vi "Actor Core.vi"(8 "error in":errorcluster, 11 "Message Logger in":refnum<class "Classic Logger.lvclass">) -> (0 "error out":errorcluster, 3 "Actor out":refnum<class "Actor.lvclass">)   [LabVIEW 2023, in "Monitored Actor.lvlib" / "Classic Logger.lvclass"]
doc: "(<B>Filename</B>: Actor Framework.lvlib:Actor.lvclass:Actor Core.vi)\n\nReceives messages to the actor, reacts to them, and initiates any error handling that may shut the actor down.\n\nDescendant classes may override this VI to append parallel tasks for the actor to complete while it handles messages. Overrides use the Call Parent Method node."
uses:
  Classic Logger.lvclass
  C:/Users/Public/Documents/Development/builds/Engine/Actor Framework.lvlibp/1abvi3w/vi.lib/ActorFramework/Actor/Actor.lvclass
  builds/Engine/Actor Framework.lvlibp/1abvi3w/vi.lib/ActorFramework/Actor/Actor.lvclass
  UI Data.ctl
  builds/Engine/Actor Framework.lvlibp/1abvi3w/vi.lib/ActorFramework/Message Enqueuer/Message Enqueuer.lvclass
  <vilib>/Utility/miscctls.llb/LVRowAndColumnTypeDef.ctl
  Classic Logger.lvclass/Classic Logger.ctl
  Monitor Data.ctl
  <vilib>/Utility/miscctls.llb/LVRowAndColumnUnsignedTypeDef.ctl
  Classic Logger Messages/Clear Log Msg/Clear Log Msg.lvclass
  Classic Logger Messages/Stop Logging Msg/Stop Logging Msg.lvclass
  builds/Engine/Actor Framework.lvlibp/1abvi3w/vi.lib/ActorFramework/Stop Msg/Stop Msg.lvclass
panel:
  in  "Actors":i32(listbox) caption="Actors Being Logged"
  in  "Stop Monitoring":bool
  in  "Log":i32(listbox)
  out "Filtered Msgs":i16
  in  "Clear Log":bool
  out "Message XML":string
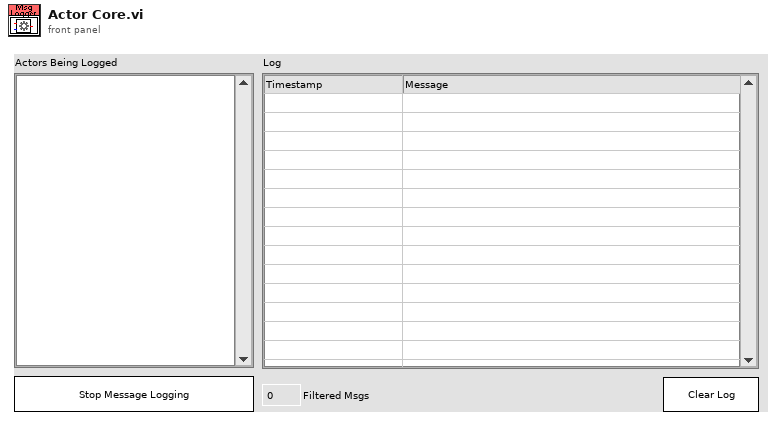
[diagram p1: front panel]
types:
  T1 = typedef "LVRowAndColumnTypeDef.ctl" = cluster{"Row":i32, "Column":i32}
  T2 = enum32{"Invalid", "Standard", "Closed", "Hidden", "Minimized", "Maximized"}
  T3 = typedef "Monitored Actor.lvlib/Classic Logger.lvclass/UI Data.ctl" = cluster{"Actors":cluster{"Q":refnum<class "Message Enqueuer.lvclass">, "Label":string}[], "Message Log":variant}
  T4 = typedef "LVRowAndColumnUnsignedTypeDef.ctl" = cluster{"Row":u32, "Column":u32}
  T5 = typedef "Monitored Actor.lvlib/Classic Logger.lvclass/Monitor Data.ctl" = cluster{"Time Stamp":timestamp, "class name":string, "Msg XML":string}
  T6 = cluster{"Q":refnum<class "Message Enqueuer.lvclass">, "Label":string}[]
  T7 = cluster{"Q":refnum<class "Message Enqueuer.lvclass">, "Label":string}
  T8 = cluster{"Actors":cluster{"Q":refnum<class "Message Enqueuer.lvclass">, "Label":string}[], "Message Log":variant}
  T9 = typedef "LVPoint32TypeDef.ctl" = cluster{"Horizontal":i32, "Vertical":i32}
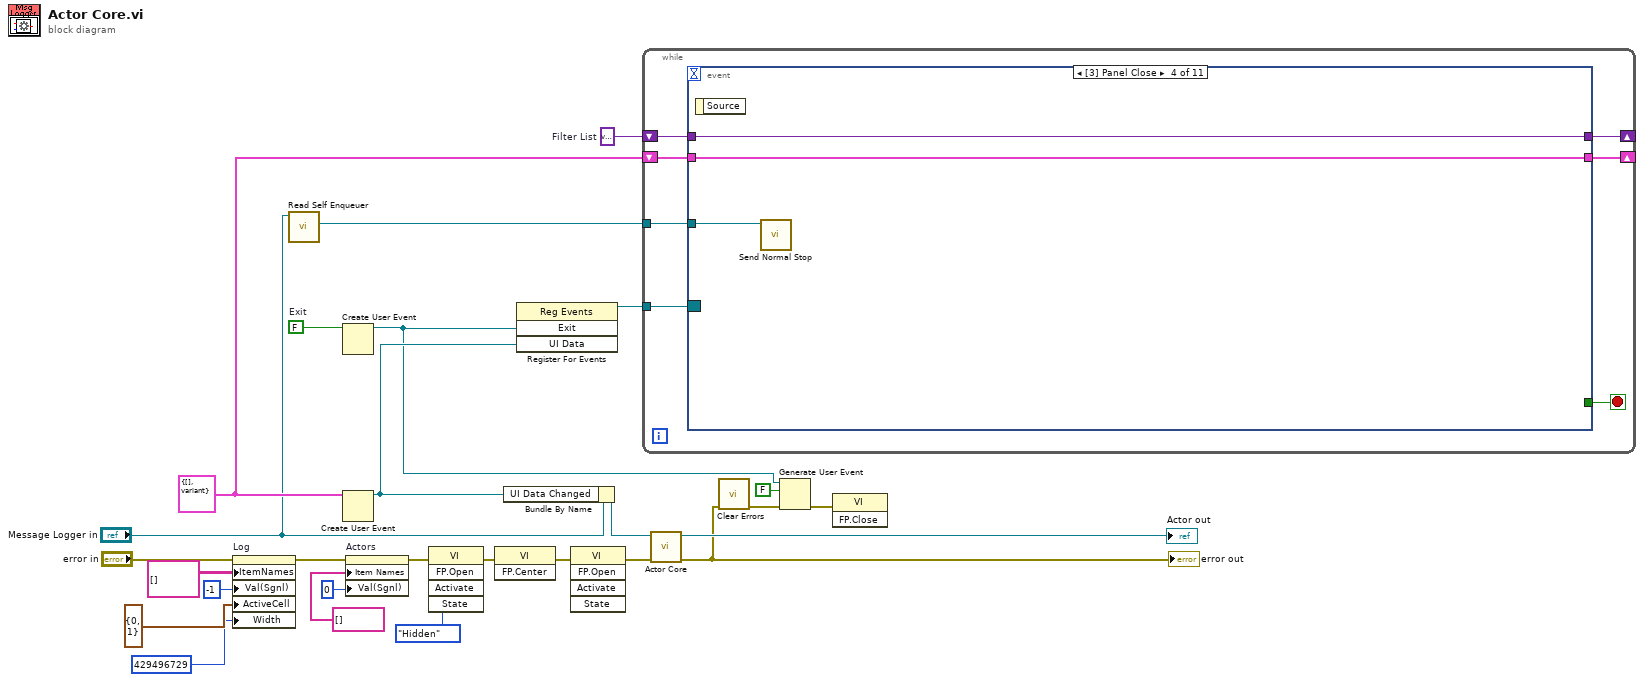
[diagram p0: block diagram]
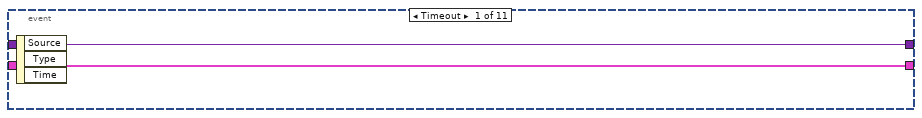
[diagram p2: hidden frame]
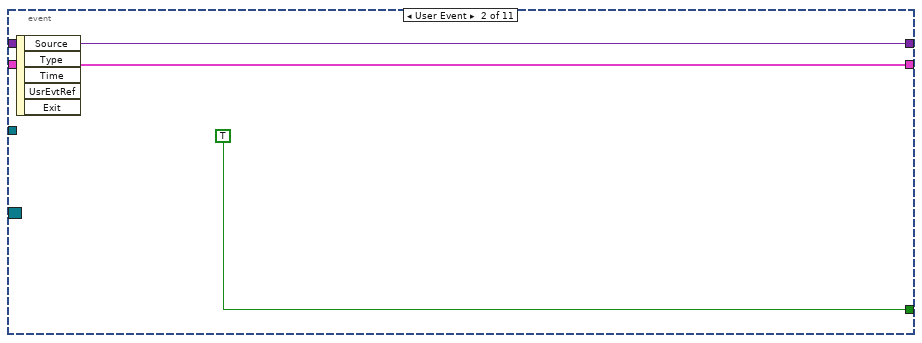
[diagram p3: hidden frame]
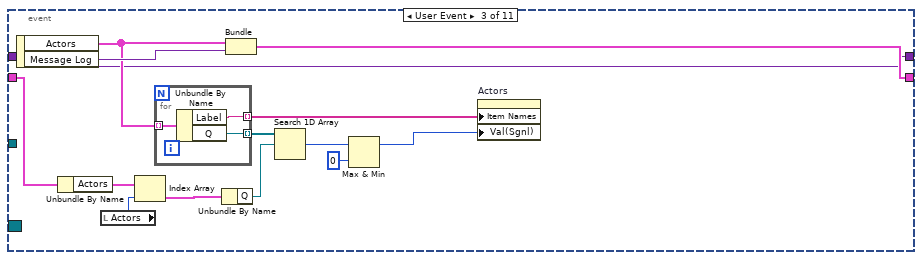
[diagram p4: hidden frame]
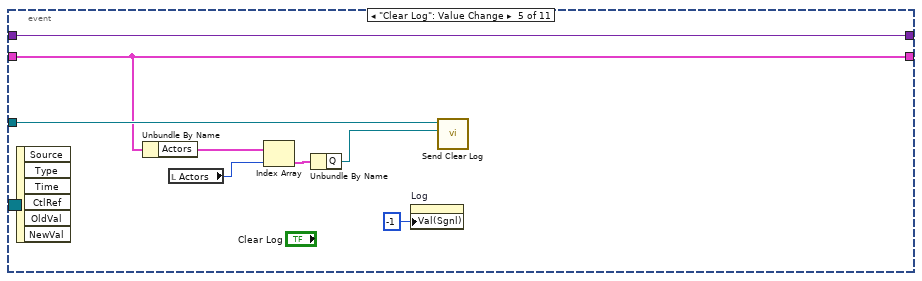
[diagram p5: hidden frame]
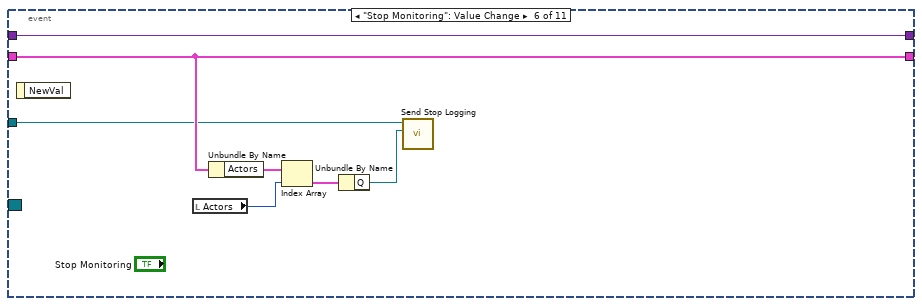
[diagram p6: hidden frame]
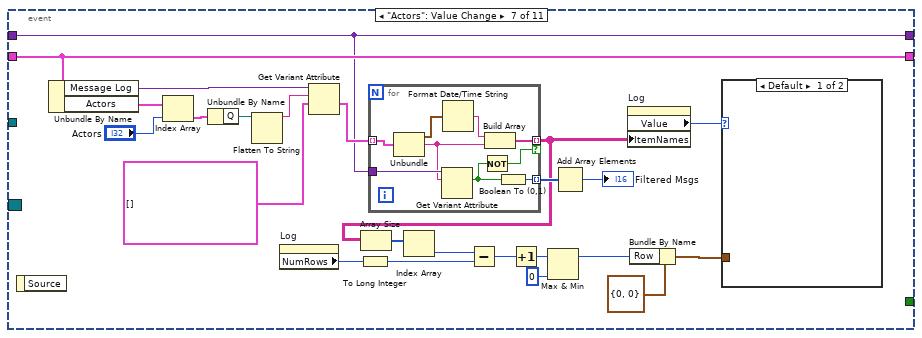
[diagram p7: hidden frame]
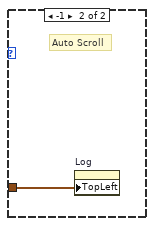
[diagram p8: hidden frame]
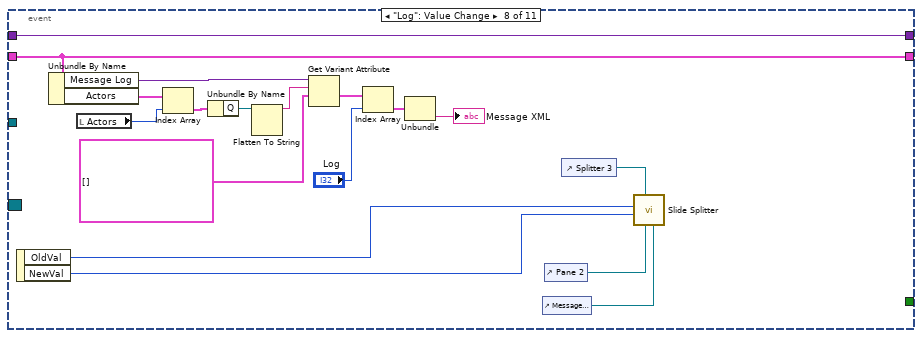
[diagram p9: hidden frame]
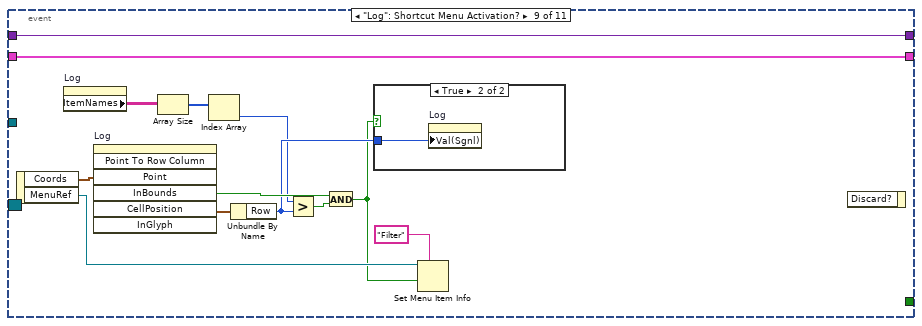
[diagram p10: hidden frame]
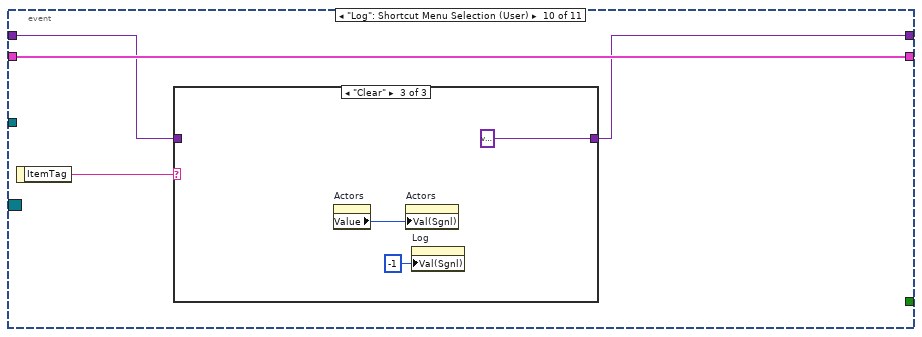
[diagram p12: hidden frame]
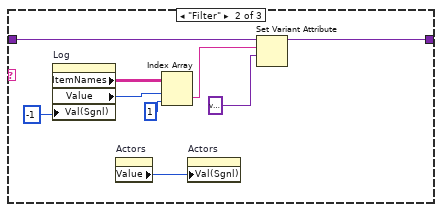
[diagram p14: hidden frame]
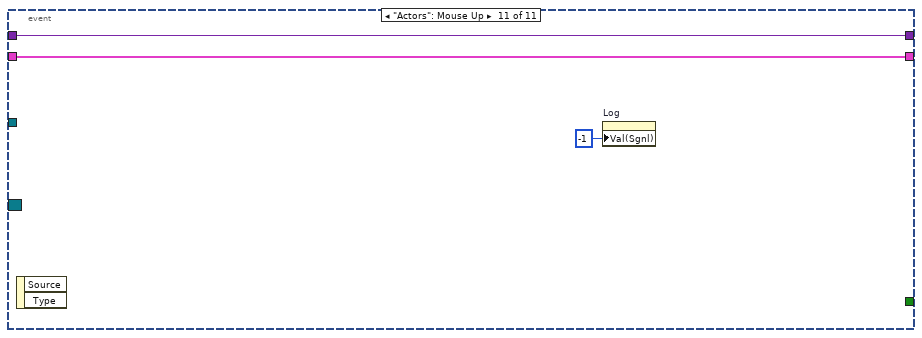
[diagram p15: hidden frame]
diagram:
  w5 = variant  # Filter List
  w21 = FALSE  # Exit
  w13 = T3 {"Actors"=[], "Message Log"=variant} ("UI Data")
  n1 = property on="Log" class="MCListbox (strict)"(error in="error in", "ItemNames"=string[][] [] ("Item Names"), "Val(Sgnl)"=-1 ("Log"), "ActiveCell"=T1 {"Row"=0, "Column"=1} ("Active Cell:Active Cell"), "Width"=u32 429496729 ("Active Cell:Cell Size:Width")) -> (error out=w15:errorcluster)  [unwired: 1 in, 1 out]
  n2 = call "Read Self Enqueuer.vi"("Actor"="Message Logger in") -> ("Self Enqueuer"=w11:refnum<class "Message Enqueuer.lvclass">)  [unwired: 10 in]
  n3 = Create User Event(user event datatype=w21) -> (user event=w18:refnum<user-event>)  [unwired: 1 in, 1 out]
  n4 = Create User Event(user event datatype=w13) -> (user event=w23:refnum<user-event>)  [unwired: 1 in, 1 out]
  n5 = property on="Actors" class="LstBox (strict)"(error in=w15, "Item Names"=string[] [], "Val(Sgnl)"=0 ("Log")) -> (error out=w9:errorcluster)  [unwired: 1 in, 1 out]
  n6 = invoke class="VI" method="FP.Open"(error in=w9, "State"=T2."Hidden") -> (error out=w8:errorcluster)  [unwired: 3 in, 4 out]
  n7 = invoke class="VI" method="FP.Center"(error in=w8) -> (error out=w7:errorcluster)  [unwired: 2 in, 2 out]
  n8 = Bundle By Name(cluster="Message Logger in", "UI Data Changed"=w23) -> (w24:refnum<class "Classic Logger.lvclass">)
  n9 = register-events(w18, w23) -> (reference out=w22:refnum<event-registration>)  [unwired: 2 in, 1 out]
  n10 = invoke class="VI" method="FP.Open"(error in=w7) -> (error out=w17:errorcluster)  [unwired: 4 in, 4 out]
  n11 = while {
    tunnel: w22 -> [w34]
    shift-right: [w31] -> _
    shift-left: w13 -> [w32]
    tunnel: w11 -> [w30]
    shift-right: [w28] -> _
    shift-left: w5 -> [w29]
    stop <- w33 stop-if-true
    n12 = event shown="[3] Panel Close" {
      selector: w34 -> [_ _ _ _ _ _ _ _ _ _ _]
      dyn-events: _ -> [_ _ _ _ _ _ _ _ _ _ _]
      timeout: _ -> [_ _ _ _ _ _ _ _ _ _ _]
      tunnel: [_ TRUE _ _ _ _ _ _ _ _ _] -> w33
      tunnel: w32 -> [w36 w38 w47 w59 w66 w74 w98 w126 w137 w144 w160]
      tunnel: [w36 w38 w53 w59 w66 w74 w98 w126 w137 w144 w160] -> w31
      tunnel: w30 -> [_ _ _ w58 w67 w69 _ _ _ _ _]
      tunnel: w29 -> [w35 w37 w40 w57 w60 w70 w80 w114 w139 w142 w159]
      tunnel: [w35 w37 w40 w57 w60 w70 w80 w114 w139 w141 w159] -> w28
      event Timeout {
        n13 = event-data() -> ()  [unwired: 1 in, 3 out]
      }
      event User Event {
        n14 = event-data() -> ()  [unwired: 1 in, 5 out]
      }
      event User Event {
        n15 = event-data() -> ("Actors"=w51:T6, "Message Log"=w52:variant)  [unwired: 1 in]
        n16 = Unbundle By Name(w47) -> ("Actors"=w46:T6)
        n17 = local read "Actors"() -> (w45:i32)
        n18 = Index Array(array=w46, index=w45) -> (element=w44:T7)
        n19 = for {
          tunnel: w51 -> [w56] mode=indexing
          tunnel: [w55] -> w50 mode=indexing
          tunnel: [w54] -> w49 mode=indexing
          n20 = Unbundle By Name(w56) -> ("Label"=w55:string, "Q"=w54:refnum<class "Message Enqueuer.lvclass">)
        }
        n21 = Unbundle By Name(w44) -> ("Q"=w43:refnum<class "Message Enqueuer.lvclass">)
        n22 = Bundle("Actors"=w51, "Message Log"=w52) -> (w53:T8)  [unwired: 1 in]
        n23 = Search 1D Array(1D array=w49, element=w43) -> (index of element=w48:i32)  [unwired: 1 in]
        n24 = Max & Min(x=w48, y=0) -> (max(x,y)=w42:i32)  [unwired: 1 out]
        n25 = property on="Actors" class="LstBox (strict)"("Item Names"=w50, "Val(Sgnl)"=w42) -> ()  [unwired: 2 in, 2 out]
      }
      event Panel Close {
        n26 = event-data() -> ()  [unwired: 1 in, 1 out]
        n27 = call "Send Normal Stop.vi"("Message Enqueuer"=w58) -> ()  [unwired: 10 in, 1 out]
      }
      event "Clear Log": Value Change {
        n28 = event-data() -> ()  [unwired: 1 in, 6 out]
        n29 = Unbundle By Name(w66) -> ("Actors"=w65:T6)
        n30 = local read "Actors"() -> (w62:i32)
        n31 = Index Array(array=w65, index=w62) -> (element=w64:T7)
        n32 = Unbundle By Name(w64) -> ("Q"=w63:refnum<class "Message Enqueuer.lvclass">)
        n33 = property on="Log" class="MCListbox (strict)"("Val(Sgnl)"=-1 ("Value (Signaling)")) -> ()  [unwired: 2 in, 2 out]
        n34 = call "Send Clear Log.vi"("Actor Q"=w63, "Message Enqueuer in"=w67) -> ()  [unwired: 8 in, 2 out]
      }
      event "Stop Monitoring": Value Change {
        n35 = event-data() -> ()  [unwired: 1 in, 1 out]
        n36 = local read "Actors"() -> (w72:i32)
        n37 = Unbundle By Name(w74) -> ("Actors"=w73:T6)
        n38 = Index Array(array=w73, index=w72) -> (element=w71:T7)
        n39 = Unbundle By Name(w71) -> ("Q"=w68:refnum<class "Message Enqueuer.lvclass">)
        n40 = call "Send Stop Logging.vi"("Q"=w68, "Message Enqueuer in"=w69) -> ()  [unwired: 8 in, 2 out]
      }
      event "Actors": Value Change {
        n41 = event-data() -> ()  [unwired: 1 in, 1 out]
        n42 = Unbundle By Name(w98) -> ("Message Log"=w95:variant, "Actors"=w97:T6)
        n43 = Index Array(array=w97, index="Actors") -> (element=w94:T7)
        n44 = Unbundle By Name(w94) -> ("Q"=w91:refnum<class "Message Enqueuer.lvclass">)
        n45 = Flatten To String(anything=w91) -> (data string=w93:string)  [unwired: 3 in, 2 out]
        n46 = property on="Log" class="MCListbox (strict)"() -> ("NumRows"=w88:u32)  [unwired: 2 in, 2 out]
        n47 = Get Variant Attribute(Variant=w95, name=w93, default value (empty Variant)=T5[] []) -> (value=w90:T5[])  [unwired: 1 in, 3 out]
        n48 = To Long Integer(number=w88) -> (32bit integer=w81:i32)
        n49 = for {
          tunnel: w90 -> [w108] mode=indexing
          tunnel: [w105] -> w77 mode=indexing if=w102
          tunnel: w80 -> [w104]
          tunnel: [w100] -> w78 mode=indexing
          n50 = Unbundle(w108) -> ("Time Stamp"=w107:timestamp, "class name"=w103:string)  [unwired: 1 out]
          n51 = Get Variant Attribute(Variant=w104, name=w103) -> (found=w101:bool)  [unwired: 2 in, 3 out]
          n52 = Format Date/Time String(seconds (now)=w107) -> (date/time string=w106:string)  [unwired: 2 in]
          n53 = Not(x=w101) -> (.not. x?=w102:bool)
          n54 = Build Array(w106, w103) -> (w105:string[])
          n55 = Boolean To (0,1)(Boolean=w101) -> (0, 1=w100:i16)
        }
        n56 = Array Size(array=w77) -> (size(s)=w89:i32[])
        n57 = Index Array(array=w89) -> (element=w76:i32)  [unwired: 1 in]
        n58 = Subtract(x=w76, y=w81) -> (x-y=w86:i32)
        n59 = Increment(x=w86) -> (x+1=w85:i32)
        n60 = Max & Min(x=w85, y=0) -> (max(x,y)=w83:i32)  [unwired: 1 out]
        n61 = Add Array Elements(numeric array=w78) -> (sum=→"Filtered Msgs":i16)
        n62 = property on="Log" class="MCListbox (strict)"("ItemNames"=w77) -> ("Value"=w75:i32)  [unwired: 2 in, 2 out]
        n63 = Bundle By Name(cluster=T4 {"Row"=0, "Column"=0} ("Top Left Visible Cell"), "Row"=w83) -> (w84:T4)
        n64 = case shown="Default" w75 {
          tunnel: w84 -> [_ w99]
          frame Default {
          }
          frame -1 {
            # "Auto Scroll"
            n65 = property on="Log" class="MCListbox (strict)"("TopLeft"=w99) -> ()  [unwired: 2 in, 2 out]
          }
        }
      }
      event "Log": Value Change {
        n66 = event-data() -> ("OldVal"=w112:i32, "NewVal"=w111:i32)  [unwired: 1 in]
        n67 = Unbundle By Name(w126) -> ("Message Log"=w124:variant, "Actors"=w125:T6)
        n68 = local read "Actors"() -> (w119:i32)
        n69 = Index Array(array=w125, index=w119) -> (element=w123:T7)
        n70 = Unbundle By Name(w123) -> ("Q"=w120:refnum<class "Message Enqueuer.lvclass">)
        n71 = Flatten To String(anything=w120) -> (data string=w122:string)  [unwired: 3 in, 2 out]
        n72 = Get Variant Attribute(Variant=w124, name=w122, default value (empty Variant)=T5[] []) -> (value=w118:T5[])  [unwired: 1 in, 3 out]
        n73 = Index Array(array=w118, index="Log") -> (element=w117:T5)
        n74 = Unbundle(w117) -> ("Msg XML"=→"Message XML":string)  [unwired: 2 out]
        n75 = control-ref of="Message XML"() -> (w109:refnum<vi>)
        n76 = control-ref of="Pane 2"() -> (w110:refnum<vi>)
        n77 = control-ref of="Splitter 3"() -> (w113:refnum<vi>)
        n78 = call "Slide Splitter.vi"("Message XML"=w109, "Hidden Pane"=w110, "Splitter"=w113, "New Value"=w111, "Old Value"=w112) -> ()  [unwired: 7 in]
      }
      event "Log": Shortcut Menu Activation? {
        n79 = event-data() -> ("Coords"=w138:T9, "MenuRef"=w129:refnum<k9>)  [unwired: 1 in]
        n80 = property on="Log" class="MCListbox (strict)"() -> ("ItemNames"=w131:string[][])  [unwired: 2 in, 2 out]
        n81 = invoke on="Log" class="MCListbox (strict)" method="Point To Row Column"("Point"=w138) -> ("InBounds"=w134:bool, "CellPosition"=w136:T1)  [unwired: 6 in, 5 out]
        n82 = Array Size(array=w131) -> (size(s)=w135:i32[])
        n83 = Index Array(array=w135) -> (element=w130:i32)  [unwired: 1 in]
        n84 = Unbundle By Name(w136) -> ("Row"=w132:i32)
        n85 = Greater?(x=w130, y=w132) -> (0:w133:bool)
        n86 = And(x=w134, y=w133) -> (x .and. y?=w128:bool)
        n87 = case shown="True" w128 {
          tunnel: w132 -> [_ w140]
          frame False {
          }
          frame True {
            n88 = property on="Log" class="MCListbox (strict)"("Val(Sgnl)"=w140) -> ()  [unwired: 2 in, 2 out]
          }
        }
        n89 = Set Menu Item Info(7:"Filter" ("item tag"), 9:w128, 11:w129) -> ()  [unwired: 4 in, 2 out]
        n90 = event-data() -> ()  [unwired: 2 in, 1 out]
      }
      event "Log": Shortcut Menu Selection (User) {
        n91 = event-data() -> ("ItemTag"=w143:string)  [unwired: 1 in]
        n92 = case shown="\"Clear\"" w143 {
          tunnel: w142 -> [w145 w154 _]
          tunnel: [w145 w153 variant ("Filter List")] -> w141
          frame Default {
          }
          frame "Filter" {
            n93 = property on="Log" class="MCListbox (strict)"("Val(Sgnl)"=-1 ("Value (Signaling)")) -> ("ItemNames"=w151:string[][], "Value"=w150:i32)  [unwired: 2 in, 2 out]
            n94 = property on="Actors" class="LstBox (strict)"() -> ("Value"=w147:i32)  [unwired: 2 in, 2 out]
            n95 = Index Array(array=w151, index (row)=w150, index (col)=1 ("disabled index (col)")) -> (element=w148:string)
            n96 = property on="Actors" class="LstBox (strict)"("Val(Sgnl)"=w147) -> ()  [unwired: 2 in, 2 out]
            n97 = Set Variant Attribute(Variant=w154, name=w148, value=variant) -> (Variant out=w153:variant)  [unwired: 1 in, 2 out]
          }
          frame "Clear" {
            n98 = property on="Actors" class="LstBox (strict)"() -> ("Value"=w156:i32)  [unwired: 2 in, 2 out]
            n99 = property on="Actors" class="LstBox (strict)"("Val(Sgnl)"=w156) -> ()  [unwired: 2 in, 2 out]
            n100 = property on="Log" class="MCListbox (strict)"("Val(Sgnl)"=-1 ("Value (Signaling)")) -> ()  [unwired: 2 in, 2 out]
          }
        }
      }
      event "Actors": Mouse Up {
        n101 = event-data() -> ()  [unwired: 1 in, 2 out]
        n102 = property on="Log" class="MCListbox (strict)"("Val(Sgnl)"=-1 ("Value (Signaling)")) -> ()  [unwired: 2 in, 2 out]
      }
    }
  }
  n103 = call-parent "Actor Core.vi"("error in"=w17, "Actor in"=w24) -> ("error out"=w20:errorcluster, "Actor out"=→"Actor out":refnum<class "Actor.lvclass">)  [unwired: 8 in]
  "error out" <- w20
  n104 = call <vilib>:"Clear Errors.vi"("error in (no error)"=w20) -> ("error out"=w19:errorcluster)  [unwired: 5 in, 1 out]
  n105 = Generate User Event(user event=w18, event data cluster=FALSE ("event data"), error in=w19) -> (error out=w1:errorcluster)  [unwired: 1 in, 1 out]
  n106 = invoke class="VI" method="FP.Close"(error in=w1) -> ()  [unwired: 2 in, 3 out]
